vi "GSIOC state machine.vi"(6 "GSIOC cmd":T1, 8 "error in (no error)":errorcluster, 9 "Command":string, 10 "ID (1)":u8=1, 11 "VISA resource name":refnum<visa-resource-name>="COM1") -> (0 "error out":errorcluster, 1 "Receive string":string, 2 "ID out":u8, 3 "Connected":bool)   [LabVIEW 2019]
uses:
  Gilson cmds.ctl
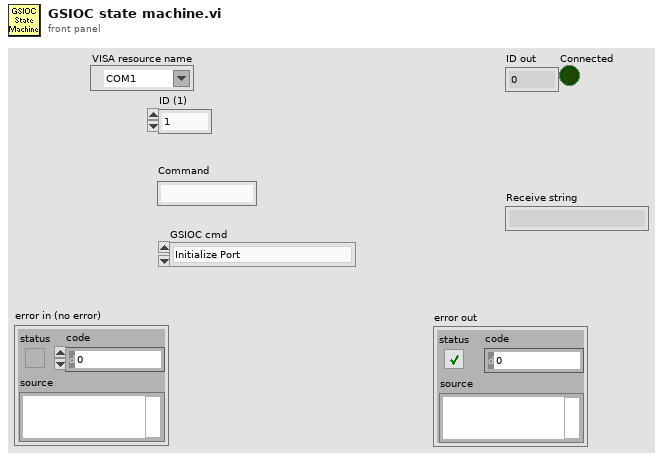
[diagram p1: front panel]
types:
  T1 = typedef "Gilson cmds.ctl" = enum16{"Initialize Port", "Immediate", "Buffered", "Connect", "Close Port"}
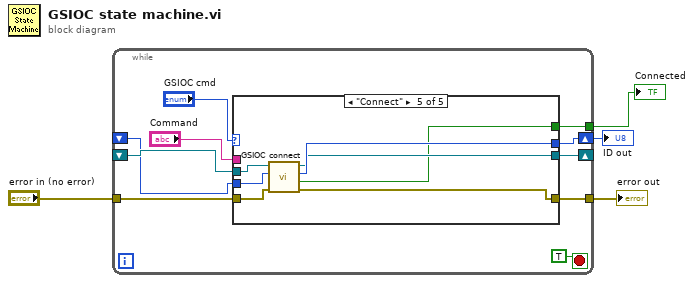
[diagram p0: block diagram]
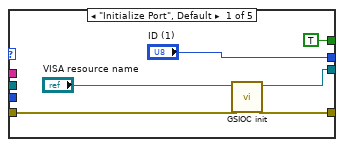
[diagram p2: hidden frame]
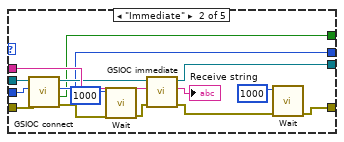
[diagram p3: hidden frame]
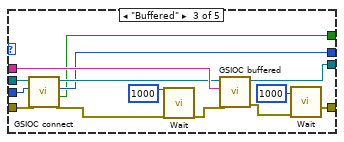
[diagram p4: hidden frame]
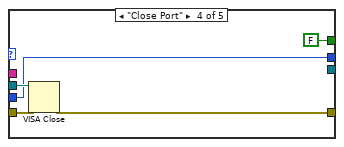
[diagram p5: hidden frame]
diagram:
  n1 = while {
    shift-right: [w12] -> _
    shift-left: _ -> [w11]
    tunnel: [w10] -> w4
    tunnel: "error in (no error)" -> [w9]
    shift-right: [w7] -> w2
    shift-left: _ -> [w6]
    tunnel: [w5] -> w1
    stop <- TRUE stop-if-true
    n2 = case shown="\"Connect\"" "GSIOC cmd" {
      tunnel: [w20 w35 w49 _ w56] -> w12
      tunnel: w11 -> [_ w31 w46 w54 w61]
      tunnel: [w19 w24 w39 w52 w58] -> w10
      tunnel: w9 -> [w18 w32 w44 w53 w59]
      tunnel: "Command" -> [_ w33 w48 _ _]
      tunnel: ["ID (1)" w28 w43 w51 w57] -> w7
      tunnel: w6 -> [_ w29 w47 w51 w60]
      tunnel: [TRUE ("Connected") w21 w36 FALSE ("Connected") w55] -> w5
      frame "Initialize Port", Default {
        n3 = call "GSIOC init.vi"("error in (no error)"=w18, "VISA resource name"="VISA resource name") -> ("error out"=w19:errorcluster, "VISA resource name out"=w20:refnum<visa-resource-name>)  [unwired: 8 in]
      }
      frame "Immediate" {
        n4 = call "GSIOC connect.vi"("error in (no error)"=w32, "ID (1)"=w29, "VISA resource name"=w31) -> ("error out"=w27:errorcluster, "Connected"=w21:bool, "ID out"=w28:u8, "VISA resource name"=w30:refnum<visa-resource-name>)  [unwired: 5 in]
        n5 = call "Wait.vi"("error in"=w27, "milliseconds to wait"=u32 1000) -> ("error out"=w26:errorcluster)  [unwired: 9 in]
        n6 = call "GSIOC immediate.vi"("error in (no error)"=w26, "Immediate command"=w33, "VISA resource name"=w30) -> ("error out"=w25:errorcluster, "Receive string"=→"Receive string":string, "VISA resource name"=w35:refnum<visa-resource-name>)  [unwired: 6 in]
        n7 = call "Wait.vi"("error in"=w25, "milliseconds to wait"=u32 1000) -> ("error out"=w24:errorcluster)  [unwired: 9 in]
      }
      frame "Buffered" {
        n8 = call "GSIOC connect.vi"("error in (no error)"=w44, "ID (1)"=w47, "VISA resource name"=w46) -> ("error out"=w42:errorcluster, "Connected"=w36:bool, "ID out"=w43:u8, "VISA resource name"=w45:refnum<visa-resource-name>)  [unwired: 5 in]
        n9 = call "Wait.vi"("error in"=w42, "milliseconds to wait"=u32 1000) -> ("error out"=w41:errorcluster)  [unwired: 9 in]
        n10 = call "GSIOC buffered.vi"("error in (no error)"=w41, "Bufferd command"=w48, "VISA resource name"=w45) -> ("error out"=w38:errorcluster, "VISA resource name out"=w49:refnum<visa-resource-name>)  [unwired: 6 in, 1 out]
        n11 = call "Wait.vi"("error in"=w38, "milliseconds to wait"=u32 1000) -> ("error out"=w39:errorcluster)  [unwired: 9 in]
      }
      frame "Close Port" {
        n12 = VISA Close(VISA resource name=w54, error in (no error)=w53) -> (error out=w52:errorcluster)
      }
      frame "Connect" {
        n13 = call "GSIOC connect.vi"("error in (no error)"=w59, "ID (1)"=w60, "VISA resource name"=w61) -> ("error out"=w58:errorcluster, "Connected"=w55:bool, "ID out"=w57:u8, "VISA resource name"=w56:refnum<visa-resource-name>)  [unwired: 5 in]
      }
    }
  }
  "error out" <- w4
  "ID out" <- w2
  "Connected" <- w1
